vi "RefreshUserEvents.vi"(8 "ErrorIn":errorcluster[](array[cluster]), 10 "Data":variant) -> (0 "ErrorOut":errorcluster[](array[cluster]))   [LabVIEW 2018]
uses:
  clUserEventDataType.ctl
  <userlib>/NIST/NISTErrorLib/NISTErrorLib.lvlib
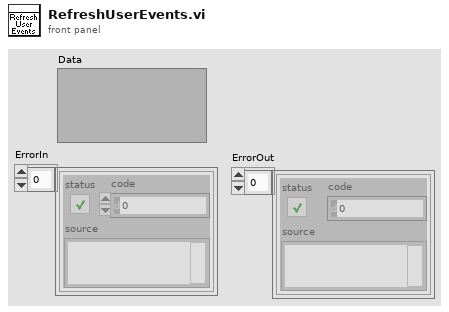
[diagram p1: front panel]
types:
  T1 = typedef "clUserEventDataType.ctl" = cluster{"Data":variant}
  T2 = typedef "clUserEvents.ctl" = cluster{"StopEvent":refnum<user-event>, "RefreshUserEvents":refnum<user-event>}
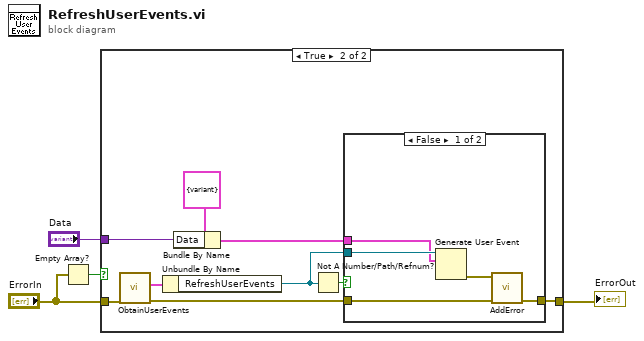
[diagram p0: block diagram]
diagram:
  n1 = Empty Array?(array="ErrorIn") -> (empty?=w4:bool)
  n2 = case shown="True" w4 {
    tunnel: "ErrorIn" -> [w5 w14]
    tunnel: [w5 w10] -> w2
    tunnel: "Data" -> [_ w6]
    frame False {
    }
    frame True {
      n3 = call "ObtainUserEvents.vi"("ErrorArray"=w14) -> ("ErrorArray"=w11:errorcluster[], "clUserEvents"=w13:T2)  [unwired: 9 in]
      n4 = Unbundle By Name(w13) -> ("RefreshUserEvents"=w9:refnum<user-event>)
      n5 = Bundle By Name(cluster=T1 {"Data"=variant} ("event data"), "Data"=w6) -> (w7:T1)
      n6 = Not A Number/Path/Refnum?(number/path/refnum=w9) -> (NaN/Path/Refnum?=w12:bool)
      n7 = case shown="False" w12 {
        tunnel: w11 -> [w17 w20]
        tunnel: [w16 w20] -> w10
        tunnel: w9 -> [w19 _]
        tunnel: w7 -> [w15 _]
        frame False {
          n8 = Generate User Event(user event=w19, event data cluster=w15) -> (error out=w18:errorcluster)  [unwired: 2 in, 1 out]
          n9 = call <userlib>:"AddError.vi"("ErrorArray"=w17, "error in (no error)"=w18) -> ("ErrorArray"=w16:errorcluster[])  [unwired: 8 in, 1 out]
        }
        frame True {
        }
      }
    }
  }
  "ErrorOut" <- w2
